vi "OR flags.vi"(11 "flags":T1[](array[typedef]) items=["O_RDONLY", "O_WRONLY", "O_RDWR"]) -> (3 "OR'ed flags":u16)   [LabVIEW 2013, in "Linux RT IPC.lvlib" / "Pipes.lvlib"]
uses:
  Pipes.lvlib
  Controls/fcntl-linux file modes.ctl
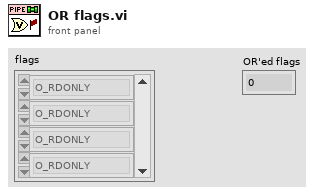
[diagram p1: front panel]
types:
  T1 = typedef "Linux RT IPC.lvlib/Pipes.lvlib/fcntl-linux file modes.ctl" = u16
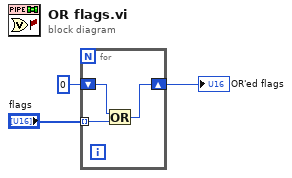
[diagram p0: block diagram]
diagram:
  n1 = for {
    tunnel: "flags" -> [w4] mode=indexing
    shift-right: [w6] -> w1
    shift-left: u16 0 -> [w5]
    n2 = Or(x=w5, y=w4) -> (x .or. y?=w6:T1)
  }
  "OR'ed flags" <- w1
